vi "XML_Load.vi"(8 "error in (no error)":errorcluster caption="错误输入（无错误）", 11 "XML File Path":path=path "E:/快盘/兰州项目资料/OPCUA XML_8.19/RT/test.xml") -> (0 "error out":errorcluster caption="错误输出", 3 "xml Data":string[](array[string]))   [LabVIEW 2017]
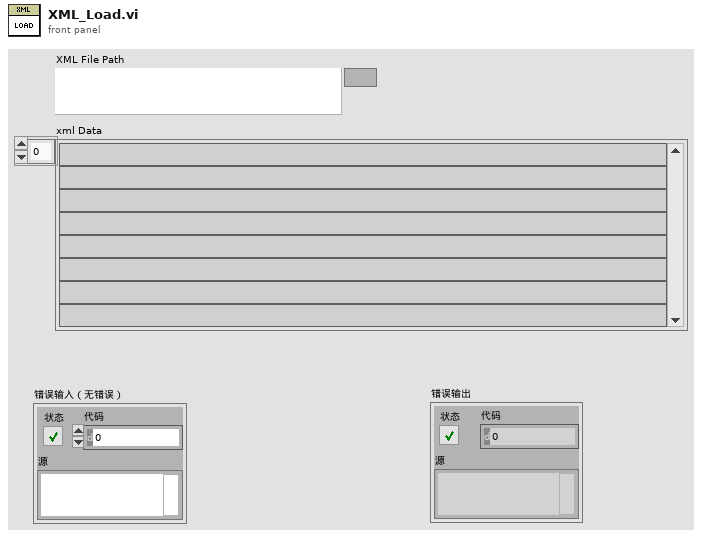
[diagram p1: front panel]
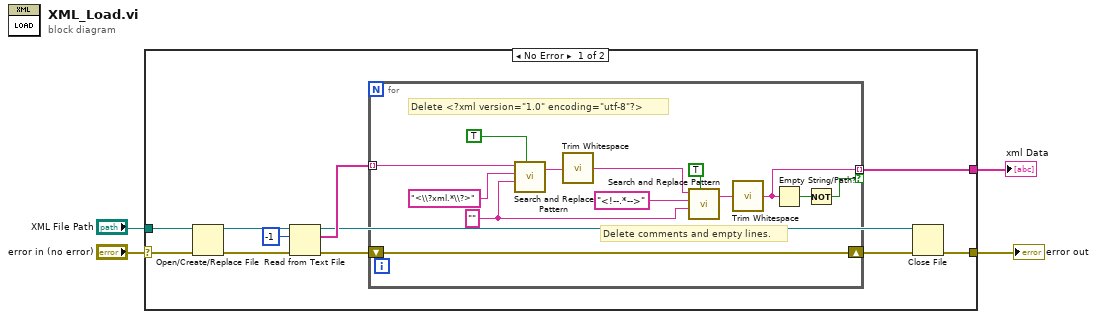
[diagram p0: block diagram]
diagram:
  n1 = case shown="No Error" "error in (no error)" {
    selector: "error in (no error)" -> [w10 w29]
    tunnel: [w9 w29] -> w3
    tunnel: "XML File Path" -> [w8 _]
    tunnel: [w5 _] -> w1
    frame No Error {
      n2 = Open/Create/Replace File(file path (use dialog)=w8, error in=w10) -> (refnum out=w15:refnum<file>, error out=w12:errorcluster)  [unwired: 4 in, 1 out]
      n3 = Read from Text File(file (use dialog)=w15, count=-1 ("计数"), error in=w12) -> (refnum out=w11:refnum<file>, text=w13:string[], error out=w7:errorcluster)  [unwired: 1 in, 1 out]
      n4 = for {
        tunnel: w13 -> [w21] mode=indexing
        tunnel: [w22] -> w5 mode=indexing if=w26
        shift-right: [w28] -> w6
        shift-left: w7 -> [w28]
        w18 = "" ("replace string (\"\")")
        # "Delete comments and empty lines."
        # "Delete <?xml version=\"1.0\" encoding=\"utf-8\"?>"
        n5 = call <vilib>:"Search and Replace Pattern.vi"("string"=w21, "regular expression (\"\")"="<\\?xml.*\\?>" ("regular expression (\"\")"), "replace string (\"\")"=w18, "replace all? (F)"=TRUE) -> ("result string"=w17:string)  [unwired: 1 in, 1 out]
        n6 = call <vilib>:"Trim Whitespace.vi"("string"=w17) -> ("trimmed string"=w16:string)  [unwired: 1 in]
        n7 = call <vilib>:"Search and Replace Pattern.vi"("string"=w16, "regular expression (\"\")"="<!--.*-->" ("regular expression (\"\")"), "replace string (\"\")"=w18, "replace all? (F)"=TRUE) -> ("result string"=w27:string)  [unwired: 1 in, 1 out]
        n8 = call <vilib>:"Trim Whitespace.vi"("string"=w27) -> ("trimmed string"=w22:string)  [unwired: 1 in]
        n9 = Empty String/Path?(string/path=w22) -> (empty?=w23:bool)
        n10 = Not(x=w23) -> (.not. x?=w26:bool)
      }
      n11 = Close File(refnum=w11, error in=w6) -> (error out=w9:errorcluster)  [unwired: 1 out]
    }
    frame Error {
    }
  }
  "error out" <- w3
  "xml Data" <- w1
